vi "Initialize Sensors C.vi"(11 "?":T1={"     Use ?\nOff       On"=[FALSE, TRUE, FALSE, TRUE], "Mode:"=FALSE, "Extra Port"="", "Hokuyo Port"="COM7", "Tx Prop  Port"="COM6", "Compass Port"="", "GPS Port"=""}) -> (3 "?":T1={"     Use ?\nOff       On"=[FALSE, TRUE, FALSE, TRUE], "Mode:"=FALSE, "Extra Port"="", "Hokuyo Port"="COM7", "Tx Prop  Port"="COM6", "Compass Port"="", "GPS Port"=""})   [LabVIEW 2014]
uses:
  <vilib>/Instr/_visa.llb/VISA Flush IO Buffer Mask.ctl
  Initialize-Standard.vi
  Hokuyo URG Series.lvlib
panel:
  in  "Checksum":bool
  in  "ID Query?":bool=TRUE
  in  "Protocol":u32(ring)=2 items=["Convert to Latest", "SCIP 1.1", "SCIP 2.0"]
  # "Initialize Sensors C"
  # "Input:"
  # "Output:"
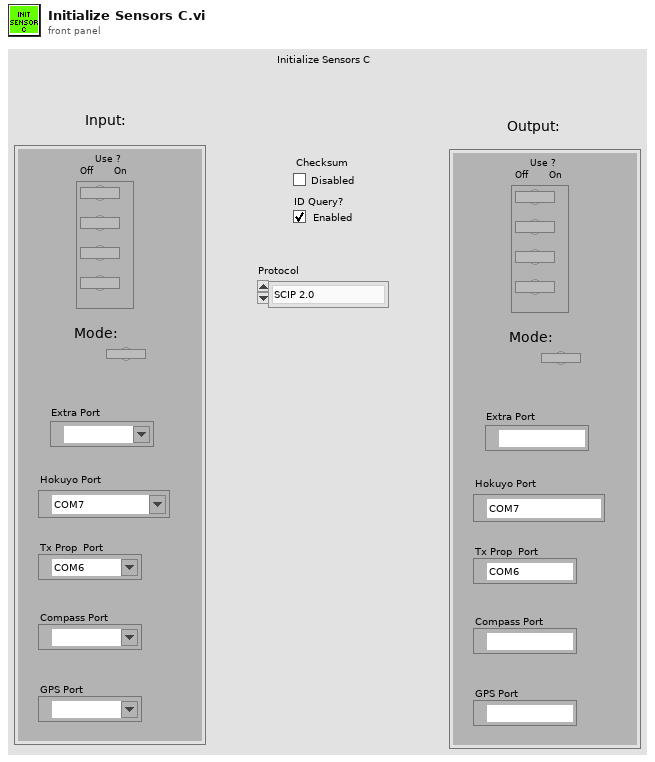
[diagram p1: front panel]
types:
  T1 = cluster{"     Use ?\nOff       On":bool[], "Mode:":bool, "Extra Port":refnum<visa-resource-name>, "Hokuyo Port":refnum<visa-resource-name>, "Tx Prop  Port":refnum<visa-resource-name>, "Compass Port":refnum<visa-resource-name>, "GPS Port":refnum<visa-resource-name>}
  T2 = typedef "VISA Flush IO Buffer Mask.ctl" = u16
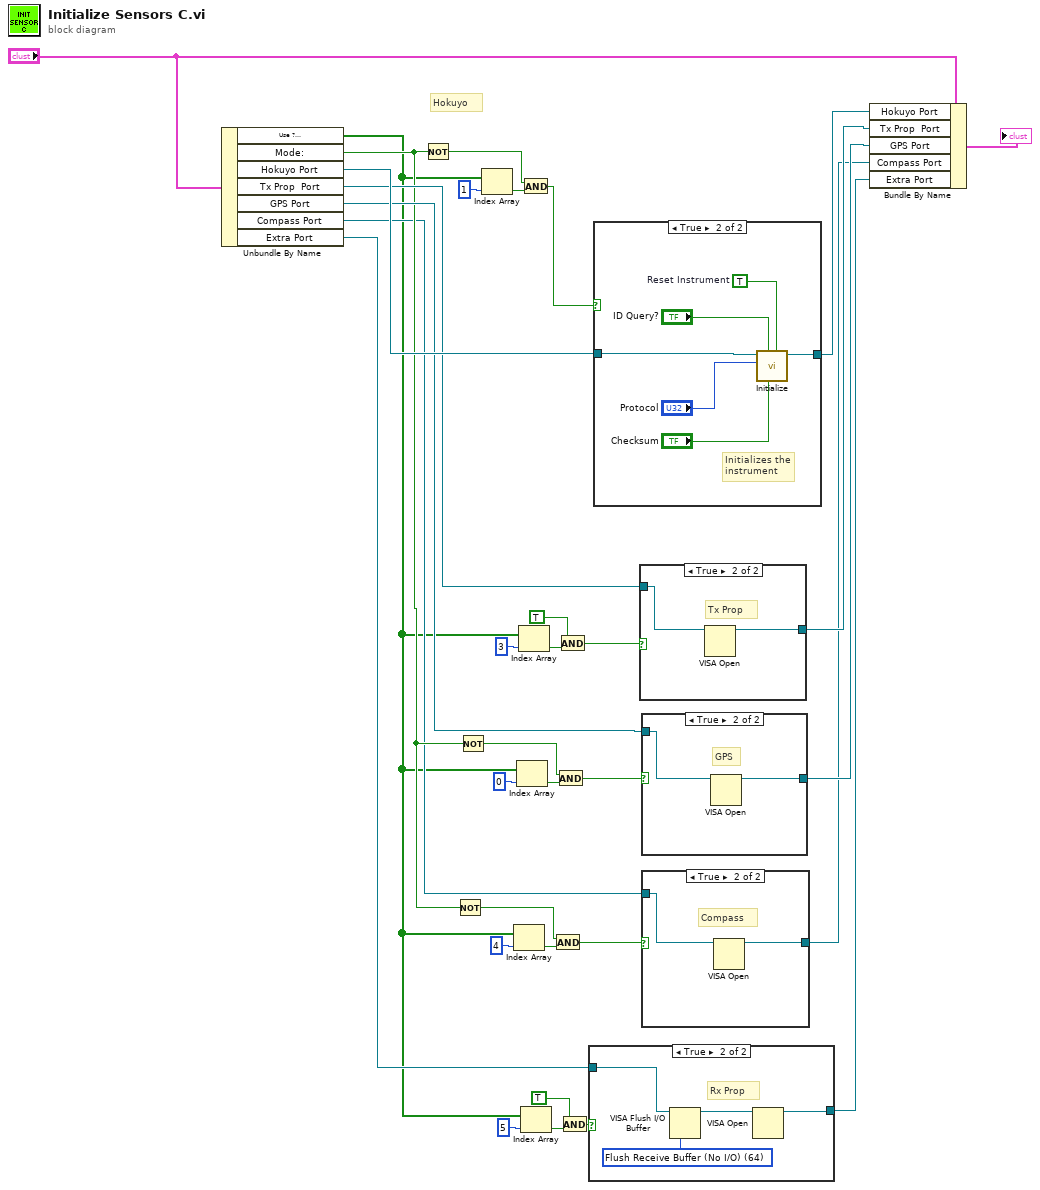
[diagram p0: block diagram]
diagram:
  # "Hokuyo"
  n1 = Unbundle By Name("?") -> ("Use ?\nOff       On"=w2:bool[], "Mode:"=w11:bool, "Hokuyo Port"=w31:refnum<visa-resource-name>, "Tx Prop  Port"=w23:refnum<visa-resource-name>, "GPS Port"=w17:refnum<visa-resource-name>, "Compass Port"=w10:refnum<visa-resource-name>, "Extra Port"=w3:refnum<visa-resource-name>)
  n2 = Not(x=w11) -> (.not. x?=w32:bool)
  n3 = Not(x=w11) -> (.not. x?=w13:bool)
  n4 = Not(x=w11) -> (.not. x?=w19:bool)
  n5 = Index Array(array=w2, index=1) -> (element=w33:bool)
  n6 = Index Array(array=w2, index=4) -> (element=w14:bool)
  n7 = Index Array(array=w2, index=0) -> (element=w20:bool)
  n8 = Index Array(array=w2, index=3) -> (element=w25:bool)
  n9 = And(x=w32, y=w33) -> (x .and. y?=w30:bool)
  n10 = Index Array(array=w2, index=5) -> (element=w6:bool)
  n11 = And(x=w13, y=w14) -> (x .and. y?=w12:bool)
  n12 = And(x=w19, y=w20) -> (x .and. y?=w18:bool)
  n13 = And(x=TRUE, y=w25) -> (x .and. y?=w24:bool)
  n14 = And(x=TRUE, y=w6) -> (x .and. y?=w5:bool)
  n15 = case shown="True" w5 {
    tunnel: w3 -> [w35 w39]
    tunnel: [w35 w37] -> w1
    frame False {
    }
    frame True {
      w36 = T2 64 items=["Flush Receive Buffer"=16, "Write Transmit Buffer to Device"=32, "Flush Receive Buffer (No I/O)"=64, "Flush Transmit Buffer"=128] ("Mask")
      # "Rx Prop"
      n16 = VISA Flush I/O Buffer(VISA resource name=w39, mask (16)=w36) -> (VISA resource name out=w38:refnum<visa-resource-name>)  [unwired: 1 in, 1 out]
      n17 = VISA Open(VISA resource name=w38) -> (VISA resource name=w37:refnum<visa-resource-name>)  [unwired: 4 in, 1 out]
    }
  }
  n18 = case shown="True" w30 {
    tunnel: w31 -> [w40 w42]
    tunnel: [w40 w41] -> w29
    frame False {
    }
    frame True {
      w44 = TRUE  # Reset Instrument
      # "Initializes the instrument"
      n19 = call-poly "Initialize.vi"("Reset? (F: No)"=w44, "Checksum (Disabled)"="Checksum", "ID Query? (Enabled)"="ID Query?", "Protocol (2: SCIP 2.0)"="Protocol", "VISA resource name"=w42) -> ("VISA resource name out"=w41:refnum<visa-resource-name>)  [unwired: 5 in, 1 out]
    }
  }
  n20 = case shown="True" w24 {
    tunnel: w23 -> [w47 w49]
    tunnel: [w47 w48] -> w22
    frame False {
    }
    frame True {
      # "Tx Prop"
      n21 = VISA Open(VISA resource name=w49) -> (VISA resource name=w48:refnum<visa-resource-name>)  [unwired: 4 in, 1 out]
    }
  }
  n22 = case shown="True" w18 {
    tunnel: w17 -> [w50 w52]
    tunnel: [w50 w51] -> w16
    frame False {
    }
    frame True {
      # "GPS"
      n23 = VISA Open(VISA resource name=w52) -> (VISA resource name=w51:refnum<visa-resource-name>)  [unwired: 4 in, 1 out]
    }
  }
  n24 = case shown="True" w12 {
    tunnel: w10 -> [w53 w55]
    tunnel: [w53 w54] -> w9
    frame False {
    }
    frame True {
      # "Compass"
      n25 = VISA Open(VISA resource name=w55) -> (VISA resource name=w54:refnum<visa-resource-name>)  [unwired: 4 in, 1 out]
    }
  }
  n26 = Bundle By Name(cluster="?", "Hokuyo Port"=w29, "Tx Prop  Port"=w22, "GPS Port"=w16, "Compass Port"=w9, "Extra Port"=w1) -> (→"?":T1)
